vi "Worker Lib Path to Name and Variant.vi"(11 "Worker Library Path":path) -> (2 "Worker Variant":string, 3 "Worker Name":string)   [LabVIEW 2022 SP3, in "FlexBlocks Support.lvlib"]
uses:
  FlexBlocks Support.lvlib
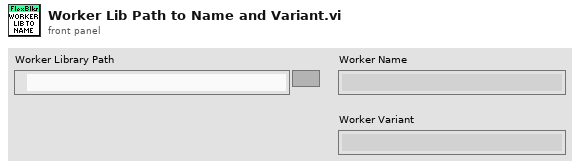
[diagram p1: front panel]
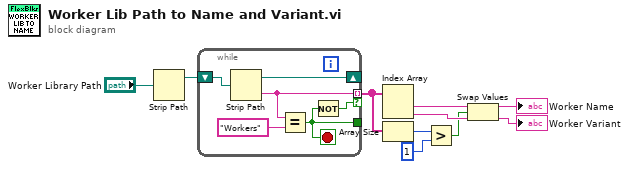
[diagram p0: block diagram]
diagram:
  n1 = Strip Path(path="Worker Library Path") -> (stripped path=w10:path)  [unwired: 1 out]
  n2 = while {
    shift-right: [w15] -> _
    shift-left: w10 -> [w16]
    tunnel: [w14] -> w8 mode=indexing if=w11
    tunnel: [w12] -> _
    stop <- w12 stop-if-true
    n3 = Strip Path(path=w16) -> (stripped path=w15:path, name=w14:string)
    n4 = Equal?(x=w14, y="Workers") -> (x = y?=w12:bool)
    n5 = Not(x=w12) -> (.not. x?=w11:bool)
  }
  n6 = Index Array(array=w8) -> (element #1=w5:string, element #2=w4:string)  [unwired: 2 in]
  n7 = Array Size(array=w8) -> (size(s)=w7:i32)
  n8 = Greater?(x=w7, y=1) -> (0:w3:bool)
  n9 = Swap Values(12:w5, 13:w3, 14:w4) -> (1:→"Worker Name":string, 3:→"Worker Variant":string)
